vi "LinearSystemSim_Update.vi"(6 "dT_Seconds":dbl=0.02, 11 "in LinearSystemSim":T1) -> (3 "out LinearSystemSim":T1)   [LabVIEW 2019, in "Trajectory_Library.lvlib"]
doc: "Creates a new LINEAR SYSTEM data cluster with the specified values. \n\n\nInputs: \n - XXX -- XXX.\n\nOutputs:\n - XXX -- XXX."
uses:
  Trajectory_Library.lvlib
  LINEAR_SYSTEM_SIM.ctl
  LINEAR_SYSTEM.ctl
  <vilib>/Analysis/Matrix/Datatypes/RealMatrix.ctl
  <vilib>/Analysis/Matrix/NI_Matrix.lvlib
panel:
  # "<States, 1>"
  # "<Outputs, 1>"
  # "<Inputs, 1>"
  # "<Outputs, 1>"
  # "<States,States>"
  # "<States,Inputs>"
  # "<Outputs,States>"
  # "<Outputs,Inputs>"
  # "<States, 1>"
  # "<Outputs, 1>"
  # "<Inputs, 1>"
  # "<Outputs, 1>"
  # "<States,States>"
  # "<States,Inputs>"
  # "<Outputs,States>"
  # "<Outputs,Inputs>"
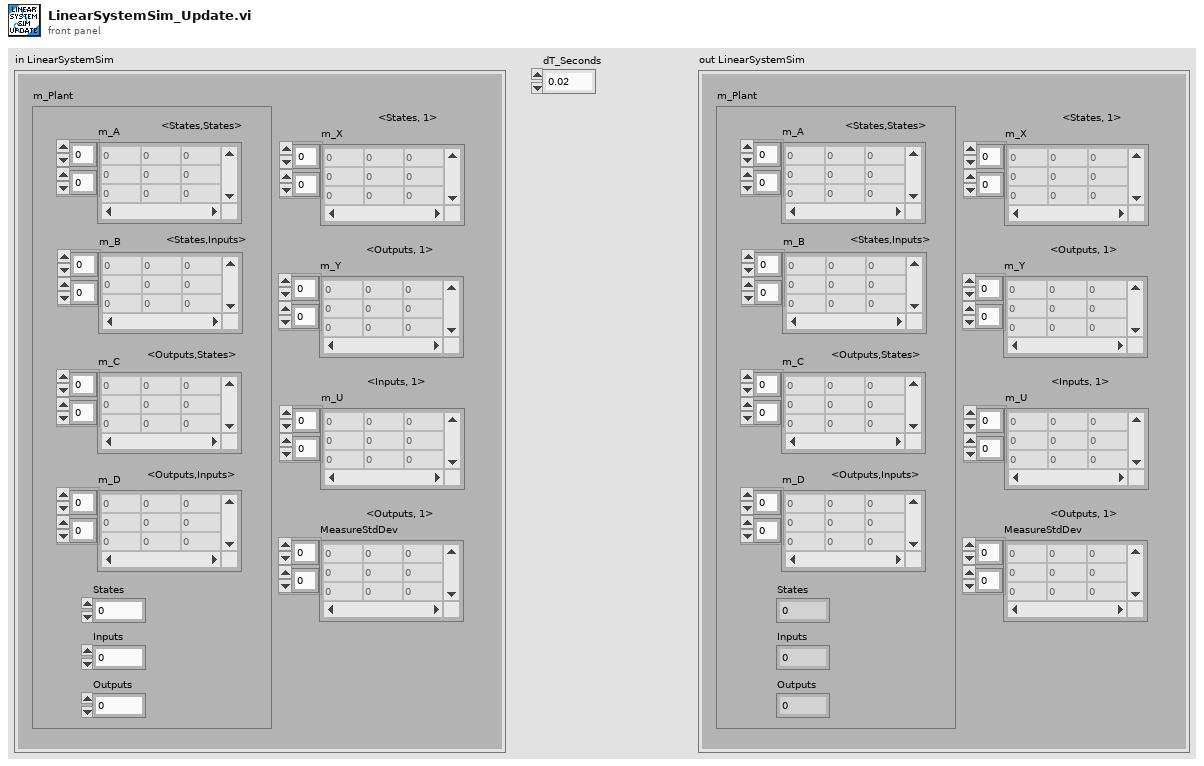
[diagram p1: front panel]
types:
  T1 = typedef "Trajectory_Library.lvlib/LINEAR_SYSTEM_SIM.ctl" = cluster{"m_Plant":T2, "m_X":T3, "m_Y":T3, "m_U":T3, "MeasureStdDev":T3}
  T2 = typedef "Trajectory_Library.lvlib/LINEAR_SYSTEM.ctl" = cluster{"m_A":T3, "m_B":T3, "m_C":T3, "m_D":T3, "States":i32, "Inputs":i32, "Outputs":i32}
  T3 = typedef "NI_Matrix.lvlib/RealMatrix.ctl" = dbl[][]
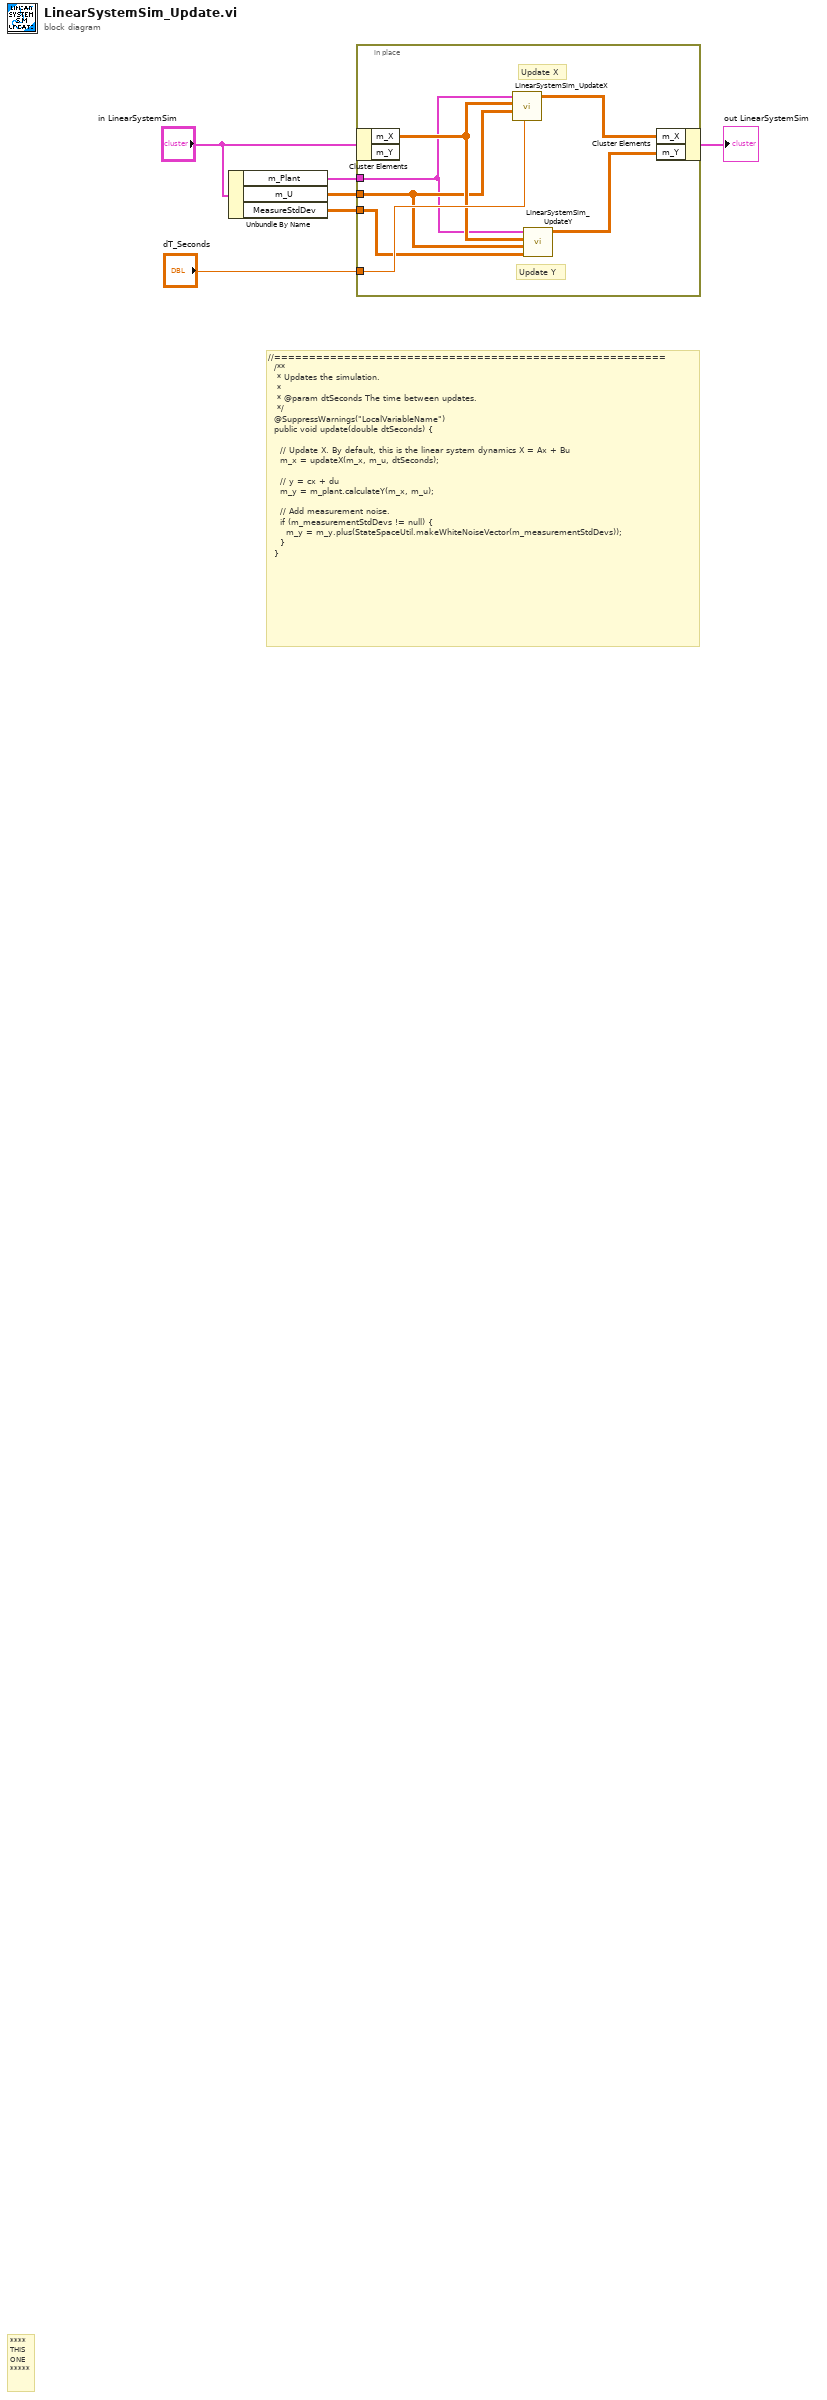
[diagram p0: block diagram]
diagram:
  # "//========================================================\n  /**\n   * Updates the simulation.\n   *\n   * @param dtSeconds The time between updates.\n   */\n  @SuppressWarnings(\"LocalVariableName\")\n  public void update(double dtSeconds) {\n\n    // Update X. By default, this is the linear system dynamics X = Ax + Bu\n    m_x = updateX(m_x, m_u, dtSeconds);\n\n    // y = cx + du\n    m_y = m_plant.calculateY(m_x, m_u);\n\n    // Add measurement noise.\n    if (m_measurementStdDevs != null) {\n      m_y = m_y.plus(StateSpaceUtil.makeWhiteNoiseVector(m_measurementStdDevs));\n    }\n  }"
  # "****\nTHIS\nONE\n*****"
  n1 = Unbundle By Name("in LinearSystemSim") -> ("m_Plant"=w6:T2, "m_U"=w5:T3, "MeasureStdDev"=w1:T3)
  n2 = in-place {
    in-place-border: w6 -> [w8]
    in-place-border: w5 -> [w10]
    in-place-border: "dT_Seconds" -> [w13]
    in-place-border: w1 -> [w7]
    # "Update Y"
    # "Update X"
    n3 = in-place-cluster #1("in LinearSystemSim") -> ("m_X"=w11:T3)  [unwired: 1 out]
    n4 = call "LinearSystemSim_UpdateX.vi"("dT_Seconds"=w13, "U"=w10, "CurrentXHat"=w11, "in LinearSystem"=w8) -> ("X"=w12:T3)  [unwired: 7 in]
    n5 = call "LinearSystemSim_UpdateY.vi"("MeasurementStdDev"=w7, "ClampedU"=w10, "X"=w11, "Linearsystem"=w8) -> ("Y"=w9:T3)  [unwired: 7 in]
    n6 = in-place-cluster #1("m_X"=w12, "m_Y"=w9) -> (→"out LinearSystemSim":T1)
  }
